vi "Get Balance.vi"(8 "error in (no error)":errorcluster, 10 "Account Number":string, 11 "Account Database in":refnum<class "Account Database.lvclass">) -> (0 "error out":errorcluster, 2 "Account Balance":string, 3 "Account Database out":refnum<class "Account Database.lvclass">)   [LabVIEW 2020, in "Account Database.lvclass"]
uses:
  Account Database.lvclass
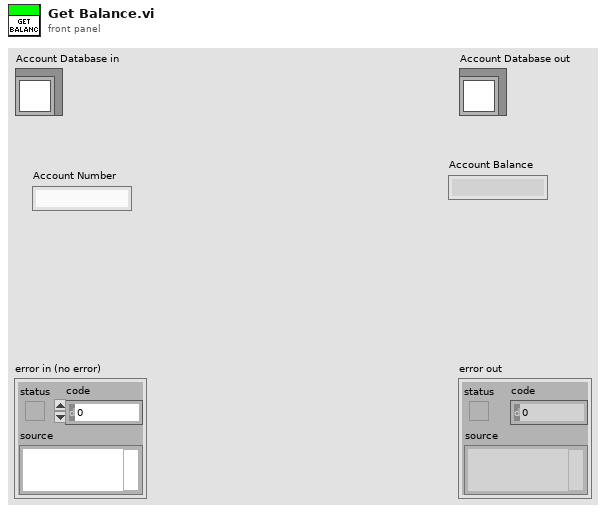
[diagram p1: front panel]
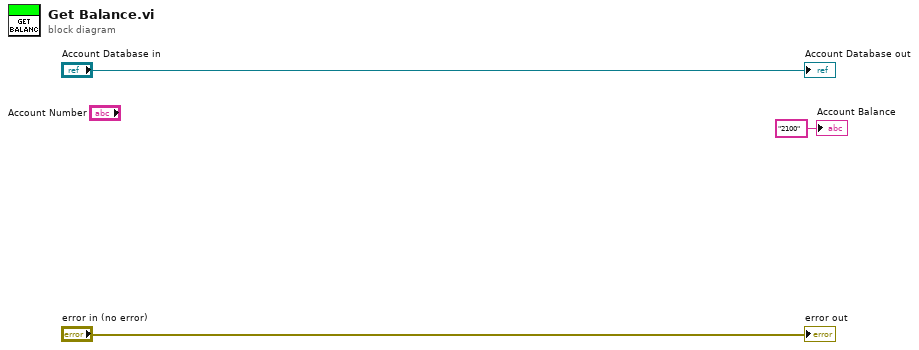
[diagram p0: block diagram]
diagram:
  "error out" <- "error in (no error)"
  "Account Database out" <- "Account Database in"
  "Account Balance" <- "2100" ("Account Balance")
